vi "CSV_Image_Data_Create.vi"(3 "error in (no error)":errorcluster, 4 "File name":string, 5 "Image path":string) -> (0 "error out":errorcluster, 1 "Image data file":path)   [LabVIEW 2024]
uses:
  <vilib>/Utility/file.llb/Write Delimited Spreadsheet (string).vi
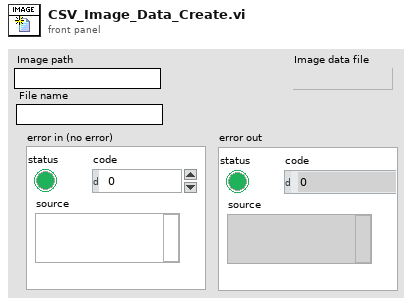
[diagram p1: front panel]
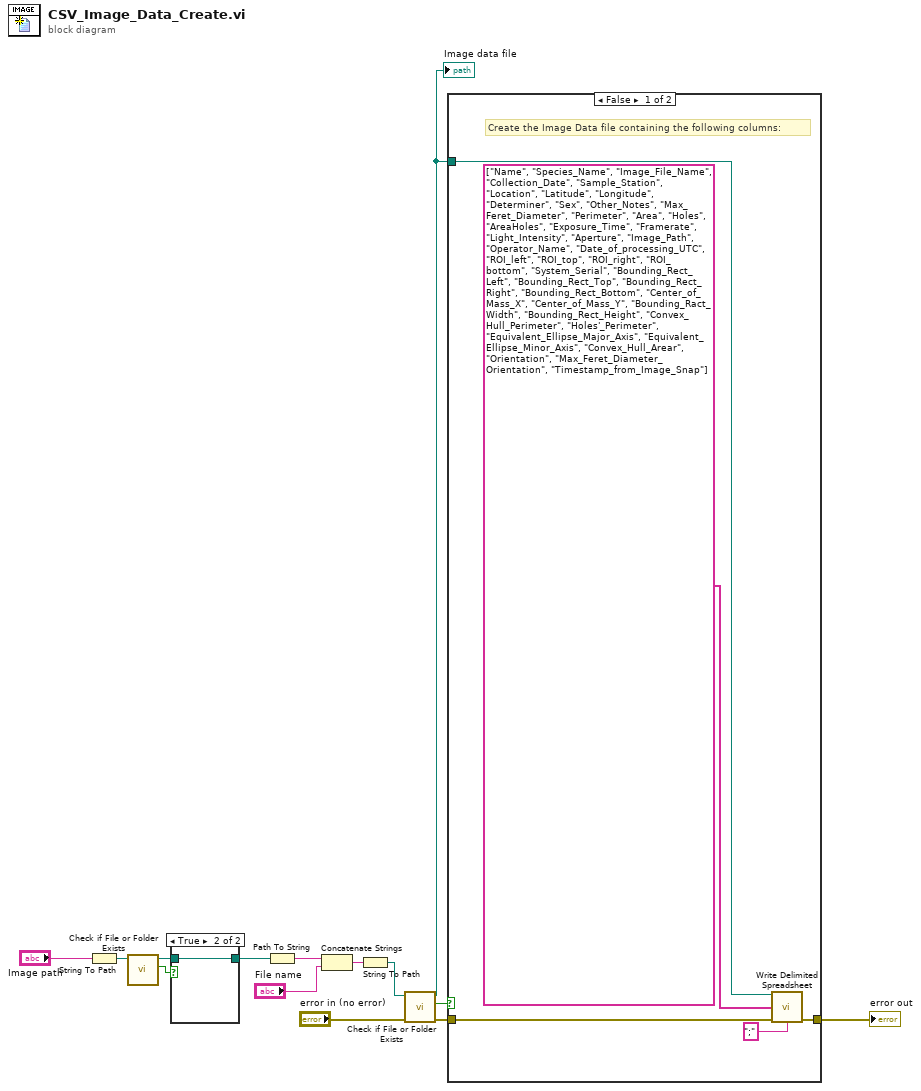
[diagram p0: block diagram]
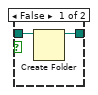
[diagram p2: hidden frame]
diagram:
  # "Create the Image Data file containing the following columns:"
  n1 = String To Path(string="Image path") -> (path=w7:path)
  n2 = call <vilib>:"Check if File or Folder Exists.vi"("path"=w7) -> ("file or folder exists?"=w6:bool, "dup path"=w5:path)  [unwired: 8 in, 1 out]
  n3 = case shown="True" w6 {
    tunnel: w5 -> [w16 w17]
    tunnel: [w15 w17] -> w4
    frame False {
      n4 = Create Folder(path (use dialog)=w16) -> (created path=w15:path)  [unwired: 2 in, 2 out]
    }
    frame True {
    }
  }
  n5 = Path To String(path=w4) -> (string=w14:string)
  n6 = Concatenate Strings(w14, "File name") -> (w13:string)
  n7 = String To Path(string=w13) -> (path=w12:path)
  n8 = call <vilib>:"Check if File or Folder Exists.vi"("error in (no error)"="error in (no error)", "path"=w12) -> ("error out"=w10:errorcluster, "file or folder exists?"=w11:bool, "dup path"=w1:path)  [unwired: 7 in]
  "Image data file" <- w1
  n9 = case shown="False" w11 {
    tunnel: w1 -> [w18 _]
    tunnel: w10 -> [w21 w23]
    tunnel: [w20 w23] -> w8
    frame False {
      n10 = call-poly <vilib>:"Write Delimited Spreadsheet.vi"("file path (dialog if empty)"=w18, "1D data"=string[] ["Name", "Species_Name", "Image_File_Name", "Collection_Date", "Sample_Station", "Location", "Latitude", "Longitude", "Determiner", "Sex", "Other_Notes", "Max_Feret_Diameter", "Perimeter", "Area", "Holes", "AreaHoles", "Exposure_Time", "Framerate", "Light_Intensity", "Aperture", "Image_Path", "Operator_Name", "Date_of_processing_UTC", "ROI_left", "ROI_top", "ROI_right", "ROI_bottom", "System_Serial", "Bounding_Rect_Left", "Bounding_Rect_Top", "Bounding_Rect_Right", "Bounding_Rect_Bottom", "Center_of_Mass_X", "Center_of_Mass_Y", "Bounding_Ract_Width", "Bounding_Rect_Height", "Convex_Hull_Perimeter", "Holes'_Perimeter", "Equivalent_Ellipse_Major_Axis", "Equivalent_Ellipse_Minor_Axis", "Convex_Hull_Arear", "Orientation", "Max_Feret_Diameter_Orientation", "Timestamp_from_Image_Snap"], "error in (no error)"=w21, "delimiter (\\t)"=";" ("delimiter (\\t)")) -> ("error out"=w20:errorcluster)  [unwired: 10 in, 1 out]
    }
    frame True {
    }
  }
  "error out" <- w8
